vi "test--system control.vi"() -> ()   [LabVIEW 2021]
panel:
  in  "String 2":string
  in  "String":string
  in  "Numeric 2":dbl
  in  "Numeric":dbl
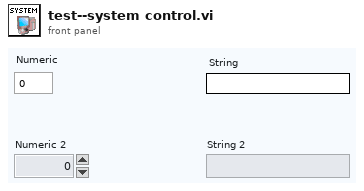
[diagram p1: front panel]
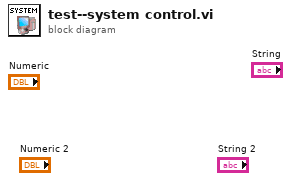
[diagram p0: block diagram]
diagram:
